vi "Do.vi"(8 "error in (no error)":errorcluster, 10 "Actor in":refnum<class "Actor.lvclass">, 11 "Process Message Msg":refnum<class "Run VI.lvclass">) -> (0 "error out":errorcluster, 2 "Actor out":refnum<class "Actor.lvclass">)   [LabVIEW 2014, in "tWorkerCommandRunner.lvlib" / "Run VI.lvclass"]
doc: "This VI delivers the message to the actor by calling the appropriate method(s) on the actor."
uses:
  Run VI.lvclass
  <vilib>/ActorFramework/Actor/Actor.lvclass
  tWorkerCommandRunner/tWorkerCommandRunner.lvclass
  Run VI.lvclass/Run VI.ctl
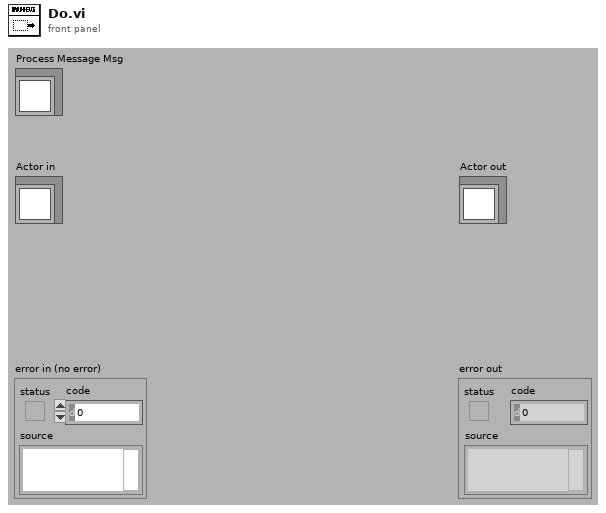
[diagram p1: front panel]
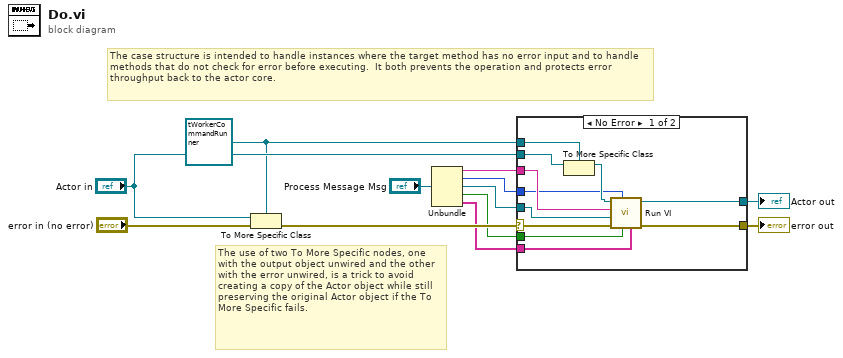
[diagram p0: block diagram]
diagram:
  w6 = refnum<class "tWorkerCommandRunner.lvclass"> refnum ("Actor in")
  # "The use of two To More Specific nodes, one with the output object unwired and the other with the error unwired, is a trick to avoid creating a copy of the Actor object while still preserving the original Actor object if the To More Specific fails."
  # "The case structure is intended to handle instances where the target method has no error input and to handle methods that do not check for error before executing.  It both prevents the operation and protects error throughput back to the actor core."
  n1 = To More Specific Class(target class=w6, reference="Actor in", error in="error in (no error)") -> (error out=w10:errorcluster)  [unwired: 1 out]
  n2 = Unbundle("Process Message Msg") -> (w5:string, w4:i32, w3:refnum<class "tBSONDocument.lvclass">, w2:bool, w1:string[])
  n3 = case shown="No Error" w10 {
    selector: w10 -> [w18 w25]
    tunnel: [w19 w25] -> w9
    tunnel: [w20 w24] -> w8
    tunnel: "Actor in" -> [w23 w24]
    tunnel: w6 -> [w22 _]
    tunnel: w5 -> [w17 _]
    tunnel: w4 -> [w16 _]
    tunnel: w3 -> [w15 _]
    tunnel: w2 -> [w14 _]
    tunnel: w1 -> [w13 _]
    frame No Error {
      n4 = To More Specific Class(target class=w22, reference=w23) -> (specific class reference=w21:refnum<class "tWorkerCommandRunner.lvclass">)  [unwired: 1 in, 1 out]
      n5 = call "Run VI.vi"("Indicator Names"=w13, "Open Front Panel"=w14, "Run Options"=w16, "error in (no error)"=w18, "VI Control Values"=w15, "VI Path"=w17, "tWorkerCommandRunner in"=w21) -> ("error out"=w19:errorcluster, "tWorkerCommandRunner out"=w20:refnum<class "tWorkerCommandRunner.lvclass">)  [unwired: 3 in]
    }
    frame Error {
      # "If type check fails, pass the original object out again."
    }
  }
  "error out" <- w9
  "Actor out" <- w8
